vi "Write Out.vi"(8 "error in (no error)":errorcluster, 10 "Out":refnum<k21>, 11 "cCRDS_new in":refnum<class "cCRDS_new.lvclass">=refnum) -> (0 "error out":errorcluster, 3 "cCRDS_new out":refnum<class "cCRDS_new.lvclass">)   [LabVIEW 2012, in "cCRDS_new.lvclass"]
uses:
  cCRDS_new.lvclass
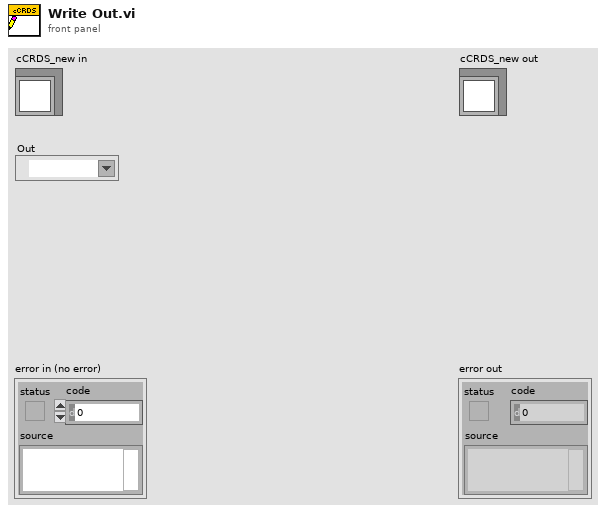
[diagram p1: front panel]
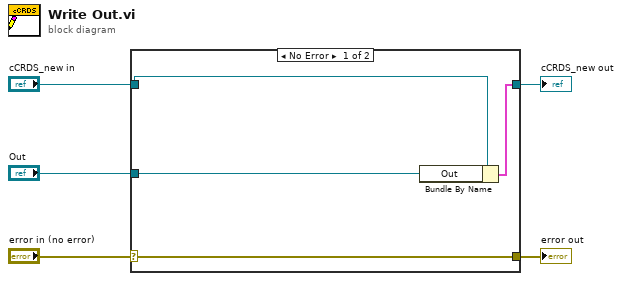
[diagram p0: block diagram]
diagram:
  n1 = case shown="No Error" "error in (no error)" {
    selector: "error in (no error)" -> [w9 w10]
    tunnel: [w9 w10] -> w4
    tunnel: [w7 w11] -> w2
    tunnel: "cCRDS_new in" -> [w8 w11]
    tunnel: "Out" -> [w6 _]
    frame No Error {
      n2 = Bundle By Name(cluster=w8, "Out"=w6) -> (w7:cluster{})
    }
    frame Error {
    }
  }
  "error out" <- w4
  "cCRDS_new out" <- w2
